vi "no timeout err.vi"(8 "error in (no error)":errorcluster) -> (0 "error out":errorcluster, 3 "Timed out?":bool)   [LabVIEW 2009]
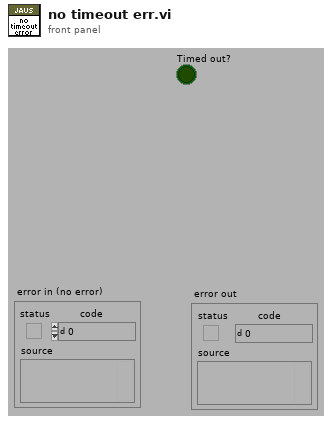
[diagram p1: front panel]
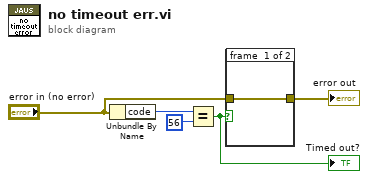
[diagram p0: block diagram]
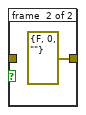
[diagram p2: hidden frame]
diagram:
  n1 = Unbundle By Name("error in (no error)") -> ("code"=w5:i32)
  n2 = Equal?(x=w5, y=56) -> (x = y?=w3:bool)
  "Timed out?" <- w3
  n3 = case shown="True" w3 {
    tunnel: "error in (no error)" -> [w6 _]
    tunnel: [w6 errorcluster {"status"=FALSE, "code"=0, "source"=""} ("error out")] -> w1
    frame #0 {
    }
    frame #1 {
    }
  }
  "error out" <- w1
